vi "DiffDrivePoseEst2_BufferDuration.vi"() -> (3 "Buffer Duration (Sec)":dbl)   [LabVIEW 2019, in "Trajectory_Library.lvlib"]
doc: "Maximum buffer duration of diff pose est 2 buffer.\n \nInputs:\n - none\n\nOutputs:\n - Buffer Duration -- double -- buffer duration (seconds)"
uses:
  Trajectory_Library.lvlib
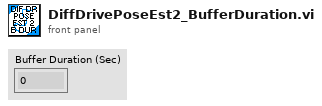
[diagram p1: front panel]
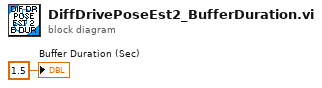
[diagram p0: block diagram]
diagram:
  "Buffer Duration (Sec)" <- 1.5 ("Buffer Duration (Sec)")
